vi "BaseActions.vi"(8 "error in (no error)":errorcluster caption="entrée d'erreur (pas d'erreur)", 11 "DNLObjectIn":refnum<class "OR77200.lvclass"> caption="DNLObject In") -> (0 "error out":errorcluster caption="sortie d'erreur", 3 "DNLObjectOut":refnum<class "OR77200.lvclass">)   [LabVIEW 2019, in "OR77200.lvclass"]
uses:
  OR77200.lvclass
  C:/Programmes Labview/LabScanV1A/DevicesClass/BaseDevice/BaseDevice.lvclass
panel:
  out "Function":string
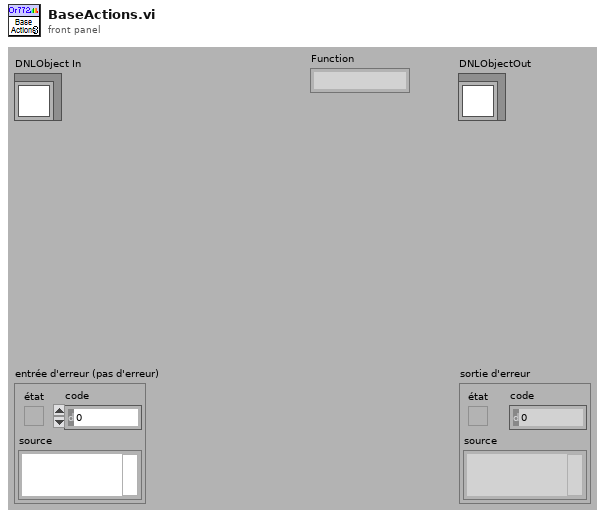
[diagram p1: front panel]
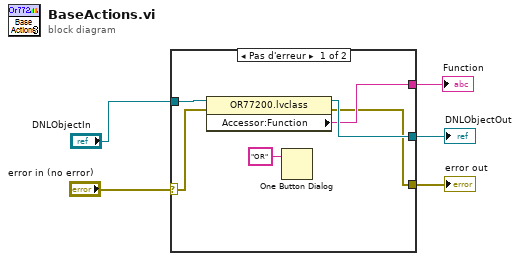
[diagram p0: block diagram]
diagram:
  n1 = case shown="Pas d'erreur" "error in (no error)" {
    selector: "error in (no error)" -> [w7 w12]
    tunnel: "DNLObjectIn" -> [w10 w13]
    tunnel: [w9 w13] -> w3
    tunnel: [w8 _] -> w2
    tunnel: [w6 w12] -> w1
    frame No Error {
      n2 = property class="OR77200.lvclass"(reference=w10, error in=w7) -> (reference out=w9:refnum<class "OR77200.lvclass">, error out=w6:errorcluster, "Accessor:Function"=w8:string)
      n3 = One Button Dialog(message="OR") -> ()  [unwired: 1 in, 1 out]
    }
    frame Error {
    }
  }
  "error out" <- w1
  "DNLObjectOut" <- w3
  "Function" <- w2
